vi "WorldRefCache.vi"(8 "Set?":bool, 11 "WorldRefIn":refnum<vi>) -> (0 "error out":errorcluster, 3 "WorldRefOut":refnum<vi>)   [LabVIEW 2014]
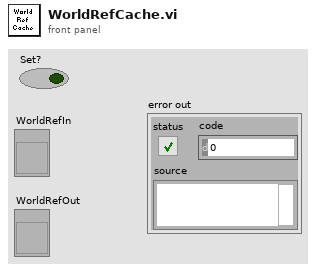
[diagram p1: front panel]
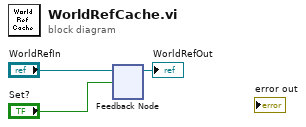
[diagram p0: block diagram]
diagram:
  n1 = feedback-in #1("WorldRefIn", "Set?") -> ()
  n2 = feedback #1() -> (→"WorldRefOut":refnum<vi>)  [unwired: 1 in]
